vi "colorgradient.vi"(11 "IntensityGraph in":refnum<vi>) -> (3 "Array":i32[][](array[numeric]))   [LabVIEW 2017]
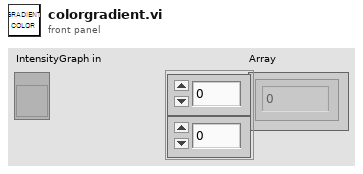
[diagram p1: front panel]
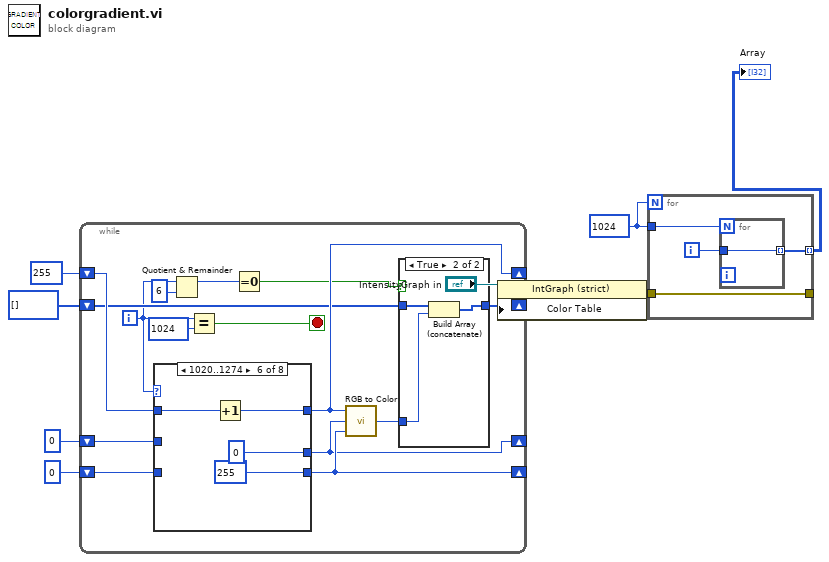
[diagram p0: block diagram]
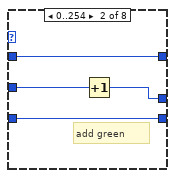
[diagram p4: hidden frame]
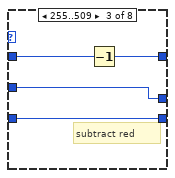
[diagram p5: hidden frame]
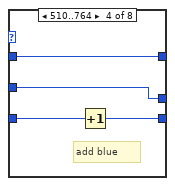
[diagram p6: hidden frame]
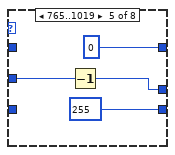
[diagram p7: hidden frame]
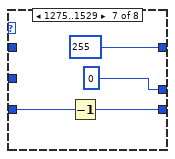
[diagram p8: hidden frame]
diagram:
  w2 = u32 1024
  n1 = while {
    shift-right: [w20] -> _
    shift-left: u8 0 ("B") -> [w22]
    shift-right: [w10] -> _
    shift-left: u8 0 ("B") -> [w23]
    shift-right: [w21] -> _
    shift-left: u8 255 ("B") -> [w24]
    shift-right: [w15] -> w8
    shift-left: u32[] [] -> [w14]
    i -> [w12]
    stop <- w11 stop-if-true
    n2 = case shown="1020..1274" w12 {
      tunnel: w24 -> [w31 w33 w39 w40 _ w51 _ w58]
      tunnel: w23 -> [w30 w35 w36 w41 w47 _ _ w57]
      tunnel: w22 -> [w29 w32 w37 w43 _ _ w53 w56]
      tunnel: [w30 w34 w36 w41 w46 u8 0 ("B") u8 0 ("B") w57] -> w10
      tunnel: [w31 w33 w38 w40 u8 0 ("B") w50 u8 255 ("B") w58] -> w21
      tunnel: [w29 w32 w37 w42 u8 255 ("B") u8 255 ("B") w52 w56] -> w20
      frame ..-1 {
      }
      frame 0..254 {
        # "add green"
        n3 = Increment(x=w35) -> (x+1=w34:u8)
      }
      frame 255..509 {
        # "subtract red"
        n4 = Decrement(x=w39) -> (x-1=w38:u8)
      }
      frame 510..764 {
        # "add blue"
        n5 = Increment(x=w43) -> (x+1=w42:u8)
      }
      frame 765..1019 {
        n6 = Decrement(x=w47) -> (x-1=w46:u8)
      }
      frame 1020..1274 {
        n7 = Increment(x=w51) -> (x+1=w50:u8)
      }
      frame 1275..1529 {
        n8 = Decrement(x=w53) -> (x-1=w52:u8)
      }
      frame 1530.. {
      }
    }
    n9 = Quotient & Remainder(x=w12, y=6) -> (x-y*floor(x/y)=w18:i32)  [unwired: 1 out]
    n10 = Equal?(x=w12, y=u32 1024 ("B")) -> (x = y?=w11:bool)
    n11 = Equal To 0?(x=w18) -> (x = 0?=w17:bool)
    n12 = call <vilib>:"RGB to Color.vi"("B"=w20, "G"=w10, "R"=w21) -> ("Color"=w16:u32)
    n13 = case shown="True" w17 {
      tunnel: w16 -> [_ w28]
      tunnel: [w25 w27] -> w15
      tunnel: w14 -> [w25 w26]
      frame False {
      }
      frame True {
        n14 = Build Array (concatenate)(w26, w28) -> (w27:u32[])
      }
    }
  }
  n15 = property on="Property Node" class="IntGraph (strict)"(reference="IntensityGraph in", "Color Table"=w8) -> (error out=w3:errorcluster)  [unwired: 1 in, 1 out]
  n16 = for {
    N: w2 -> [_]
    tunnel: w2 -> [w62]
    tunnel: [w61] -> w9 mode=indexing
    tunnel: w3 -> [w59]
    tunnel: [w59] -> _
    i -> [w60]
    n17 = for {
      N: w62 -> [_]
      tunnel: [w63] -> w61 mode=indexing
      tunnel: w60 -> [w63]
    }
  }
  "Array" <- w9
